vi "RIF_RII_filter.vi"() -> ()   [LabVIEW 2018]
uses:
  <vilib>/measure/maspectr.llb/FFT Spectrum (Mag-Phase) for 1 Chan.vi
  <vilib>/measure/macond.llb/IIR Filter for 1 Chan.vi
  <vilib>/measure/macond.llb/FIR Filter for 1 Chan.vi
  <vilib>/Analysis/NI_AALBase.lvlib
  <vilib>/measure/NI_MABase.lvlib
  <vilib>/measure/NI_MAPro.lvlib
panel:
  out "Waveform Graph 7":waveform(dbl)(graph)
  out "Waveform Graph 6":waveform(dbl)(graph)
  out "Waveform Graph 5":cluster{"f0":dbl, "df":dbl, "magnitude":dbl[]}(graph)
  out "Waveform Graph 4":cluster{"f0":dbl, "df":dbl, "magnitude":dbl[]}(graph)
  out "Waveform Graph 3":cluster{"f0":dbl, "df":dbl, "magnitude":dbl[]}(graph)
  out "Waveform Graph 2":cluster{"f0":dbl, "df":dbl, "magnitude":dbl[]}(graph)
  out "Result of Filter IIR":waveform(dbl)[](graph)
  out "Result of Filter FIR":waveform(dbl)[](graph)
  out "Phase H(w) FIR":cluster{"f0":dbl, "df":dbl, "Phase H(w)":dbl[]}(graph)
  out "Phase H(w) IIR":cluster{"f0":dbl, "df":dbl, "Mag H(w)":dbl[]}(graph)
  out "Magni H(w) IIR":cluster{"f0":dbl, "df":dbl, "Mag H(w)":dbl[]}(graph)
  in  "?":T1={"Lower SB"=200.0, "Upper SB"=0.0, "Lower PB"=100.0, "Upper PB"=0.0, "Type"=enum."Lowpass", "#Taps"=50, "Topology"=enum."FIR by Specification"} {"Lower PB" format="%0.2p"; "Upper PB" format="%0.2p"; "Lower SB" format="%0.2p"; "Upper SB" format="%0.2p"}
  in  "?":T2={"PB Ripple"=1.0, "SB Attenuation"=60.0, "Lower Fc"=100.0, "Upper Fc"=200.0, "Type"=enum."Lowpass", "Order"=1, "Topology"=enum."Butterworth"} {"Lower Fc" format="%0.2p"; "Upper Fc" format="%0.2p"; "PB Ripple" format="%0.2f"; "SB Attenuation" format="%0.2f"}
  out "Magni H(w) FIR":cluster{"f0":dbl, "df":dbl, "Mag H(w)":dbl[]}(graph)
  in  "Boolean":bool
  in  "nbr de signaux":dbl=1.0
  in  "stop":bool
  out "Waveform Graph":waveform(dbl)(graph)
  in  "Amplitude":dbl
  in  "Paramétre de siganl 2":T3={"Fréquence Echantioll"=1000.0, "nombre des echantionnage"=1000.0}
  in  "Paramétre de siganl":T4={"Amplitude"=1.0, "frequence"=15.0, "signal type"=enum."Sine Wave"}
  # "Bruit"
  # "IIR filter specifications"
  # "FIR filter specifications"
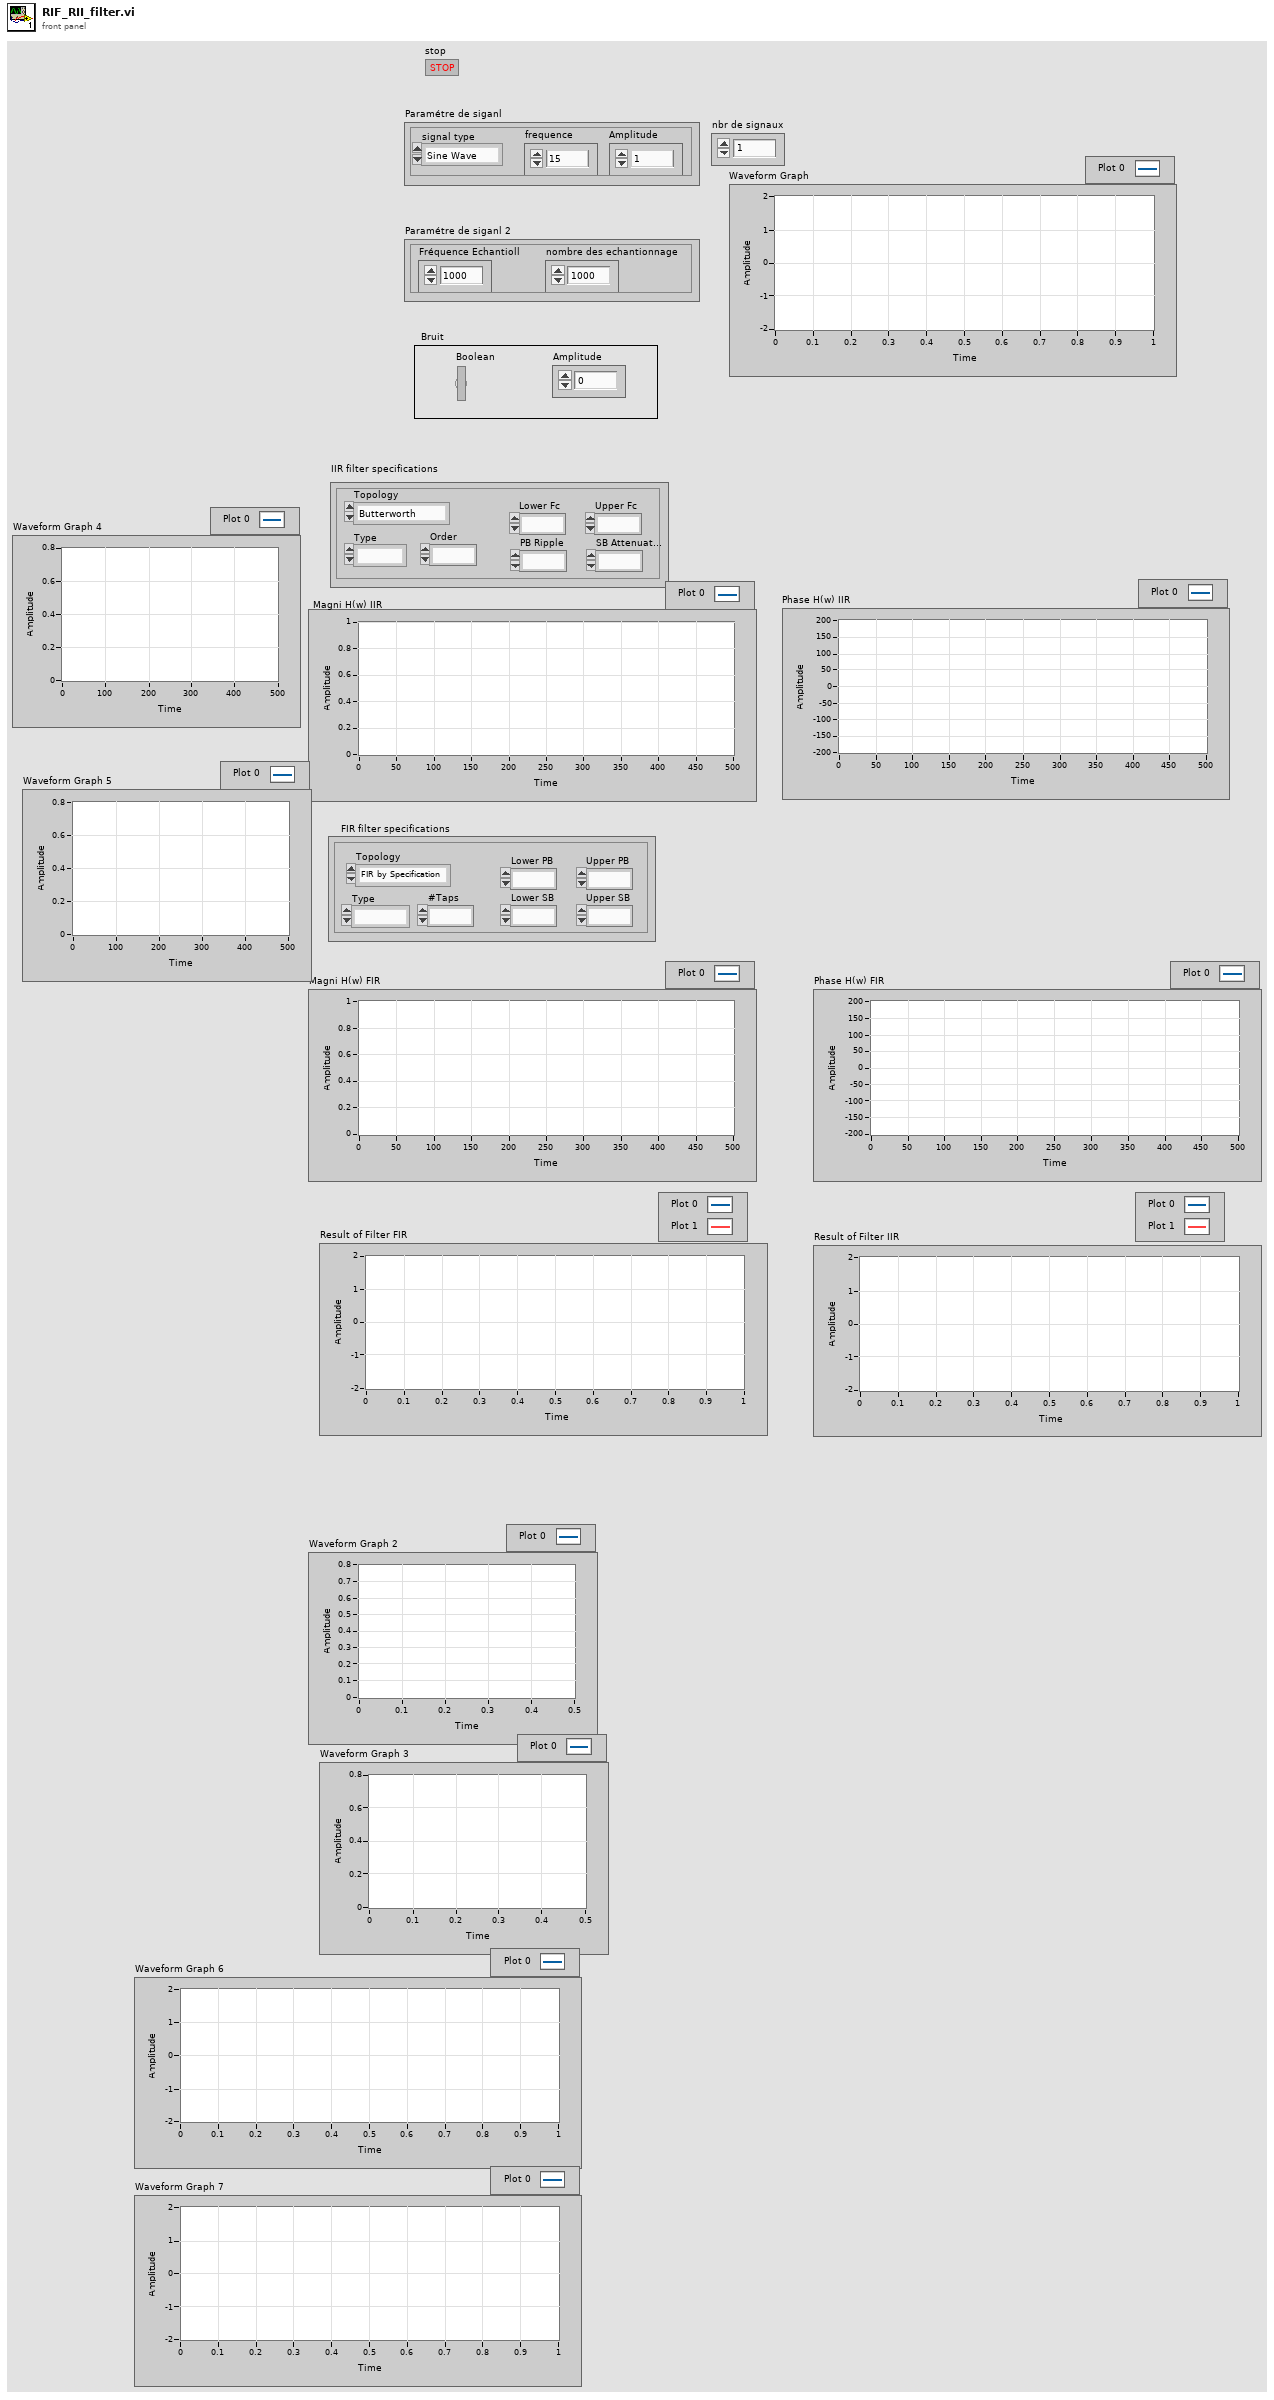
[diagram p1: front panel]
types:
  T1 = cluster{"Lower SB":dbl, "Upper SB":dbl, "Lower PB":dbl, "Upper PB":dbl, "Type":enum16{"Lowpass", "Highpass", "Bandpass", "Bandstop"}, "#Taps":i32, "Topology":enum16{"Off", "FIR by Specification", "Equi-ripple FIR", "Windowed FIR"}}
  T2 = cluster{"PB Ripple":dbl, "SB Attenuation":dbl, "Lower Fc":dbl, "Upper Fc":dbl, "Type":enum16{"Lowpass", "Highpass", "Bandpass", "Bandstop"}, "Order":i32, "Topology":enum16{"Off", "Butterworth", "Chebyshev", "Inverse Chebyshev", "Elliptic", "Bessel"}}
  T3 = cluster{"Fréquence Echantioll":dbl, "nombre des echantionnage":dbl}
  T4 = cluster{"Amplitude":dbl, "frequence":dbl, "signal type":enum16{"Sine Wave", "Triangle Wave", "Square Wave", "Sawtooth Wave"}}
  T5 = enum16{"Sine Wave", "Triangle Wave", "Square Wave", "Sawtooth Wave"}
  T6 = cluster{"magnitude H(w)":cluster{"f0":dbl, "df":dbl, "Mag H(w)":dbl[]}, "phase H(w)":cluster{"f0":dbl, "df":dbl, "Phase H(w)":dbl[]}, "order":i32}
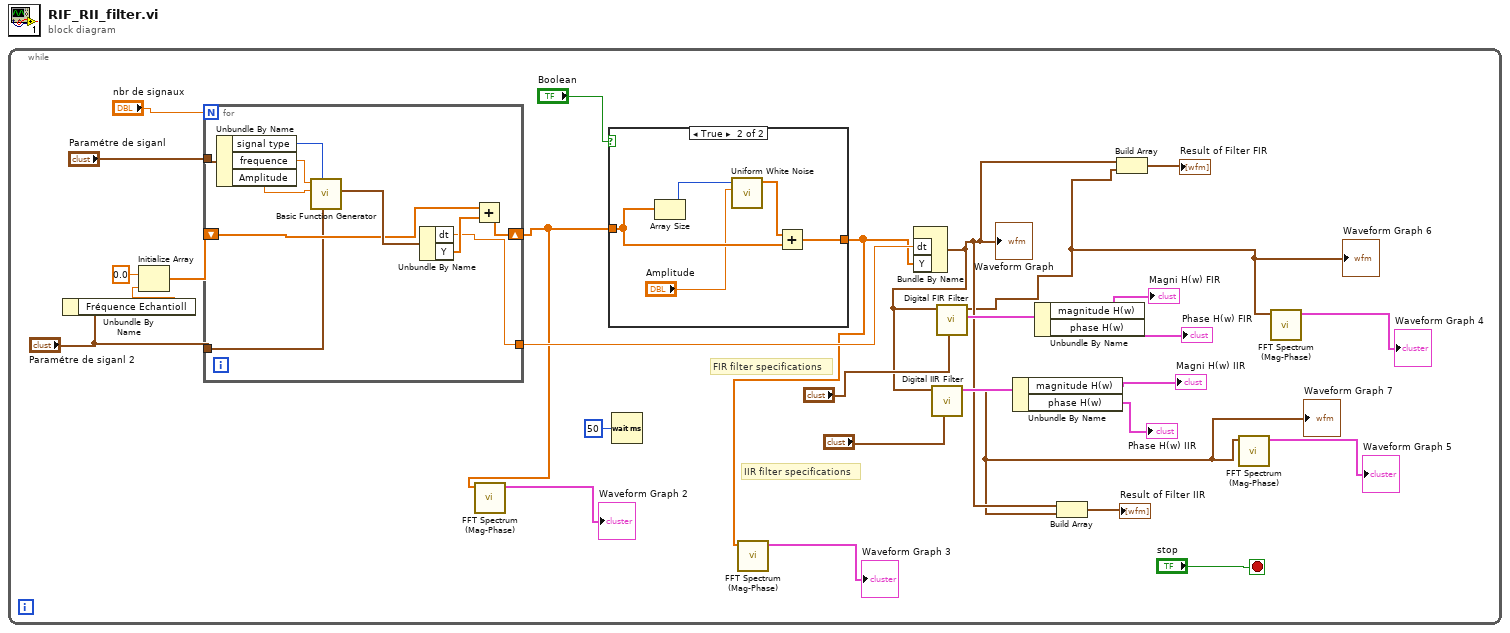
[diagram p0: block diagram]
diagram:
  n1 = while {
    stop <- "stop" stop-if-true
    # "FIR filter specifications"
    # "IIR filter specifications"
    n2 = Unbundle By Name("Paramétre de siganl 2") -> ("Fréquence Echantioll"=w27:dbl)
    n3 = Initialize Array(0.0 ("element"), w27) -> (w29:dbl[])
    n4 = for {
      N: "nbr de signaux" -> [_]
      shift-right: [w43] -> w8
      shift-left: w29 -> [w42]
      tunnel: "Paramétre de siganl 2" -> [w41]
      tunnel: [w40] -> w25
      tunnel: "Paramétre de siganl" -> [w36]
      n5 = Unbundle By Name(w36) -> ("signal type"=w39:T5, "frequence"=w38:dbl, "Amplitude"=w37:dbl)
      n6 = call <vilib>:"Basic Function Generator.vi"("sampling info"=w41, "signal type"=w39, "amplitude"=w37, "frequency"=w38) -> ("signal out"=w45:waveform(dbl))  [unwired: 5 in, 2 out]
      n7 = Unbundle By Name(w45) -> ("dt"=w40:dbl, "Y"=w44:dbl[])
      n8 = Add(x=w42, y=w44) -> (x+y=w43:dbl[])
    }
    n9 = call-poly <vilib>:"FFT Spectrum (Mag-Phase).vi"("time signal"=w8) -> ("magnitude"=→"Waveform Graph 2":cluster{"f0":dbl, "df":dbl, "magnitude":dbl[]})  [unwired: 6 in, 4 out]
    n10 = case shown="True" "Boolean" {
      tunnel: w8 -> [w30 w33]
      tunnel: [w30 w31] -> w6
      frame False {
      }
      frame True {
        n11 = Array Size(array=w33) -> (size(s)=w35:i32)
        n12 = call <vilib>:"Uniform White Noise.vi"("amplitude"="Amplitude", "samples"=w35) -> ("uniform white noise"=w34:dbl[])  [unwired: 8 in, 1 out]
        n13 = Add(x=w34, y=w33) -> (x+y=w31:dbl[])
      }
    }
    n14 = Wait (ms)(milliseconds to wait=u32 50) -> ()  [unwired: 1 out]
    n15 = call-poly <vilib>:"FFT Spectrum (Mag-Phase).vi"("time signal"=w6) -> ("magnitude"=→"Waveform Graph 3":cluster{"f0":dbl, "df":dbl, "magnitude":dbl[]})  [unwired: 6 in, 4 out]
    n16 = Bundle By Name("dt"=w25, "Y"=w6) -> (w9:waveform(dbl))  [unwired: 1 in]
    "Waveform Graph" <- w9
    n17 = call-poly <vilib>:"Digital IIR Filter.vi"("IIR filter specifications"="?", "signal in"=w9) -> ("filter information"=w17:T6, "signal out"=w1:waveform(dbl))  [unwired: 7 in, 1 out]
    "Waveform Graph 7" <- w1
    n18 = call-poly <vilib>:"Digital FIR Filter.vi"("FIR filter specifications"="?", "signal in"=w9) -> ("filter information"=w14:T6, "signal out"=w2:waveform(dbl))  [unwired: 7 in, 1 out]
    "Waveform Graph 6" <- w2
    n19 = Unbundle By Name(w17) -> ("magnitude H(w)"=→"Magni H(w) IIR":cluster{"f0":dbl, "df":dbl, "Mag H(w)":dbl[]}, "phase H(w)"=→"Phase H(w) IIR":cluster{"f0":dbl, "df":dbl, "Phase H(w)":dbl[]})
    n20 = Unbundle By Name(w14) -> ("magnitude H(w)"=→"Magni H(w) FIR":cluster{"f0":dbl, "df":dbl, "Mag H(w)":dbl[]}, "phase H(w)"=→"Phase H(w) FIR":cluster{"f0":dbl, "df":dbl, "Phase H(w)":dbl[]})
    n21 = Build Array(w9, w1) -> (→"Result of Filter IIR":waveform(dbl)[])
    n22 = Build Array(w9, w2) -> (→"Result of Filter FIR":waveform(dbl)[])
    n23 = call-poly <vilib>:"FFT Spectrum (Mag-Phase).vi"("time signal"=w1) -> ("magnitude"=→"Waveform Graph 5":cluster{"f0":dbl, "df":dbl, "magnitude":dbl[]})  [unwired: 6 in, 4 out]
    n24 = call-poly <vilib>:"FFT Spectrum (Mag-Phase).vi"("time signal"=w2) -> ("magnitude"=→"Waveform Graph 4":cluster{"f0":dbl, "df":dbl, "magnitude":dbl[]})  [unwired: 6 in, 4 out]
  }
